vi "MainRunExp.vi"() -> ()   [LabVIEW 2019, in "MotorPID.lvlib"]
uses:
  MotorPID.lvlib
  RunState.ctl
  <vilib>/Platform/TimedLoop/XDataNode/timing_clust.ctl
  <vilib>/Platform/TimedLoop/XDataNode/nitl_modes.ctl
  <vilib>/Platform/TimedLoop/XDataNode/wakeup.ctl
  <vilib>/myRIO/Common/Instrument Driver Framework/myRIO v1.0/UART/vis/myRIO v1.0 Close UART.vi
  <vilib>/addons/control/pid/pid.llb/PID (DBL).vi
  <vilib>/myRIO/Common/Instrument Driver Framework/Utilities/vis/FPGA Ref Manager.vi
  <vilib>/myRIO/Common/Instrument Driver Framework/myRIO v1.0/myRIO v1.0 Reset FPGA.vi
  <vilib>/myRIO/Common/Instrument Driver Framework/myRIO v1.0/IRQ/vis/myRIO v1.0 IRQ Info FGV.vi
  <vilib>/myRIO/Common/Instrument Driver Framework/myRIO v1.0/IRQ/vis/myRIO v1.0 Timer IRQ Info FGV.vi
  <vilib>/myRIO/Common/Instrument Driver Framework/myRIO v1.0/IRQ/vis/myRIO v1.0 ISR Agent.vi
  <vilib>/myRIO/Instrument Drivers/Utilities/vis/Reset Index.vi
  <vilib>/myRIO/Common/Instrument Driver Framework/myRIO v1.0/Resource Manager/vis/myRIO v1.0 Block Write Resource Manager.vi
  <vilib>/Platform/TimedLoop/XDataNode/XDataNode.xnode
  <vilib>/myRIO/Instrument Drivers/Utilities/Utilities.lvlib
  <vilib>/addons/control/pid/NI_PID_pid.lvlib
  <vilib>/Platform/TimedLoop/XDataNode/XDNodeRunTimeDep.lvlib
  <vilib>/ptbypt/NI_PtbyPt.lvlib
panel:
  out "State":u16(ring) items=["StickReset", "MotorReset", "MotorHome", "RunUp", "Runing", "Exit"]
  out "Waveform Chart":T1(graph)
  in  "Setpoint(deg)":dbl(knob) scale=80.0..-80.0
  out "error out":errorcluster
  out "Position(deg)":dbl(knob) scale=80.0..-80.0
  in  "Reset":bool
  in  "Stop Button":bool
  out "MotorResetPOS":dbl[](array[numeric])
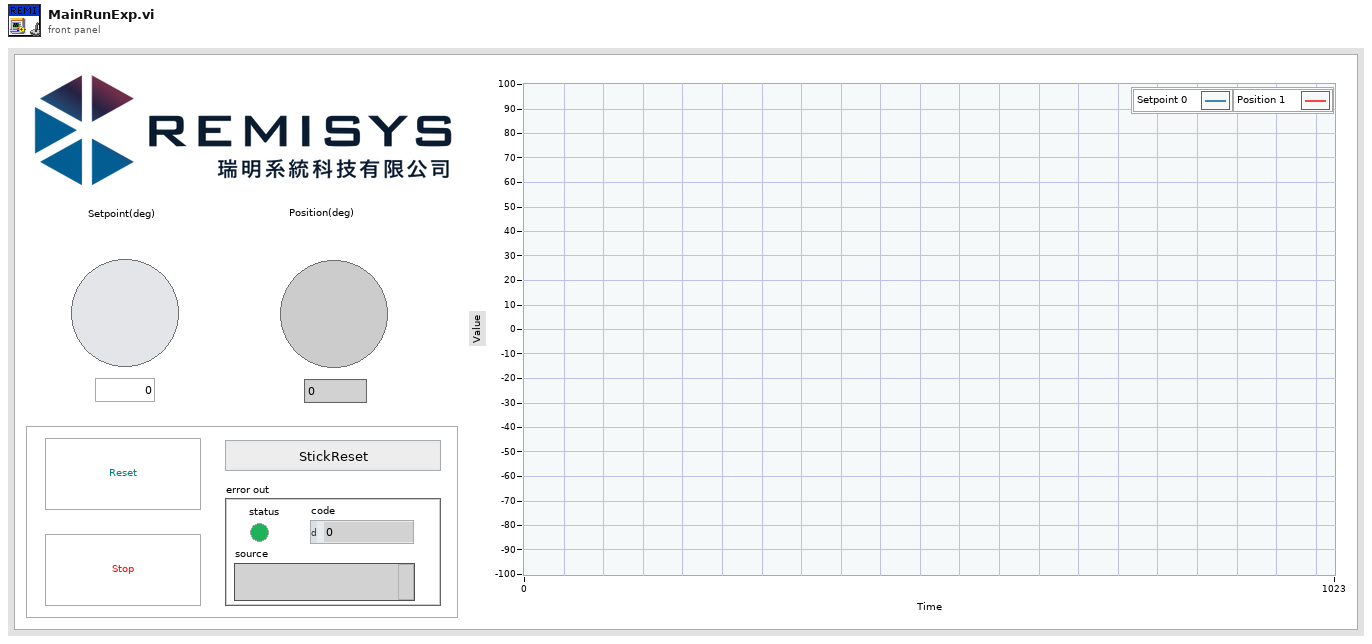
[diagram p1: front panel]
types:
  T1 = cluster{"Setpoint(deg)":dbl, "PresentPOS(deg)":dbl}
  T2 = typedef "MotorPID.lvlib/RunState.ctl" = enum16{"StickReset", "MotorReset", "MotorHome", "RunUp", "Runing", "Exit"}
  T3 = typedef "XDNodeRunTimeDep.lvlib/timing_clust.ctl" = cluster{"Expected End [f-1]":u64, "Actual End [f-1]":u64, "Finished Late? [f-1]":bool, "Expected End [i-1]":u64, "Actual End [i-1]":u64, "Finished Late? [i-1]":bool, "Expected Start [i]":u64, "Actual Start [i]":u64, "Expected Start [f]":u64, "Actual Start [f]":u64, "Source Name":string, "Structure Name":string, "Period":i64, "Deadline":i64, "Offset":i64, "Start":i64, "Priority":i32, "Timeout":i32, "Mode":T4, "Wakeup Reason":T5, "Error":errorcluster, "Source Type":string, "Secondary Source Type":string, "Global End Time":u64, "Global Start Time":u64, "Frame Duration":u64, "Iteration Duration":u64, "Assigned CPU":i32, "I/O Scan Engine Mode":u32}
  T4 = typedef "XDNodeRunTimeDep.lvlib/nitl_modes.ctl" = enum32{"No Change", "Process missed periods, maintain original phase", "Discard missed periods, maintain original phase", "Process missed periods, ignore original phase", "Discard missed periods, ignore original phase"}
  T5 = typedef "XDNodeRunTimeDep.lvlib/wakeup.ctl" = enum32{"Normal", "Aborted", "Asynchronous wakeup", "Timing source error", "Timed loop error", "Timeout"}
  T6 = cluster{"proportional gain (Kc)":dbl, "integral time (Ti, min)":dbl, "derivative time (Td, min)":dbl}
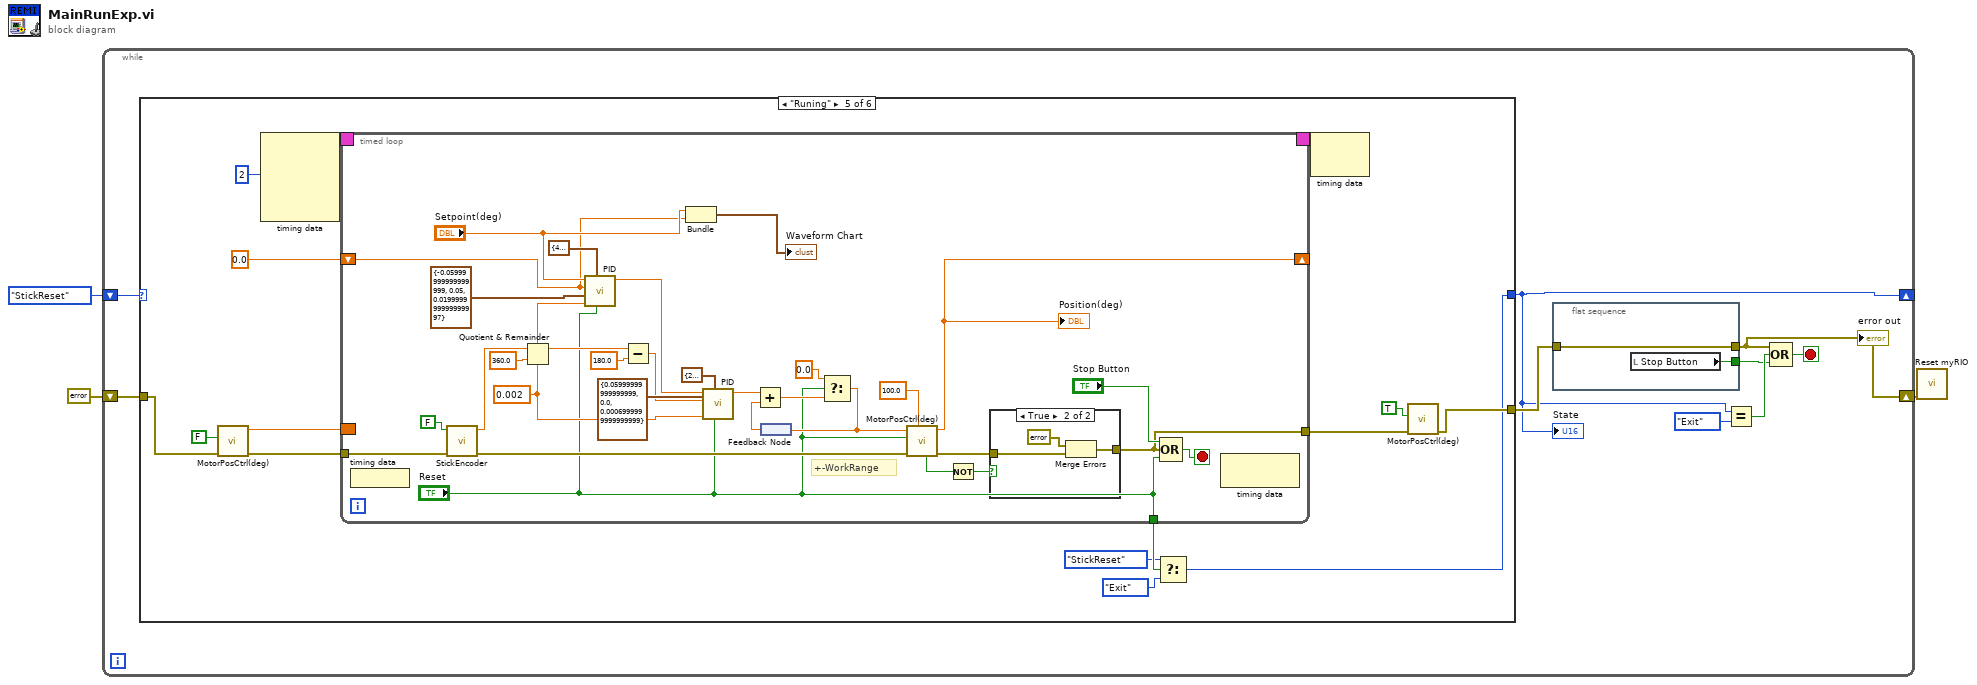
[diagram p0: block diagram]
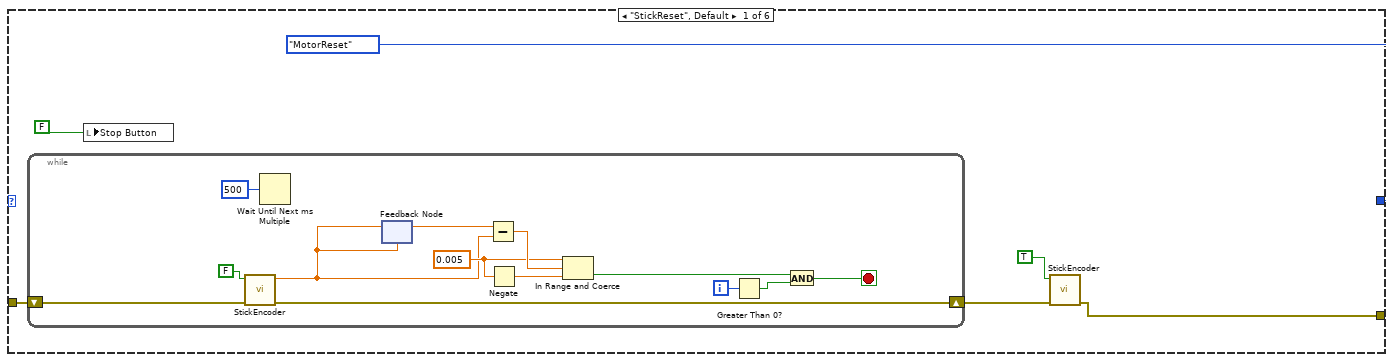
[diagram p2: hidden frame]
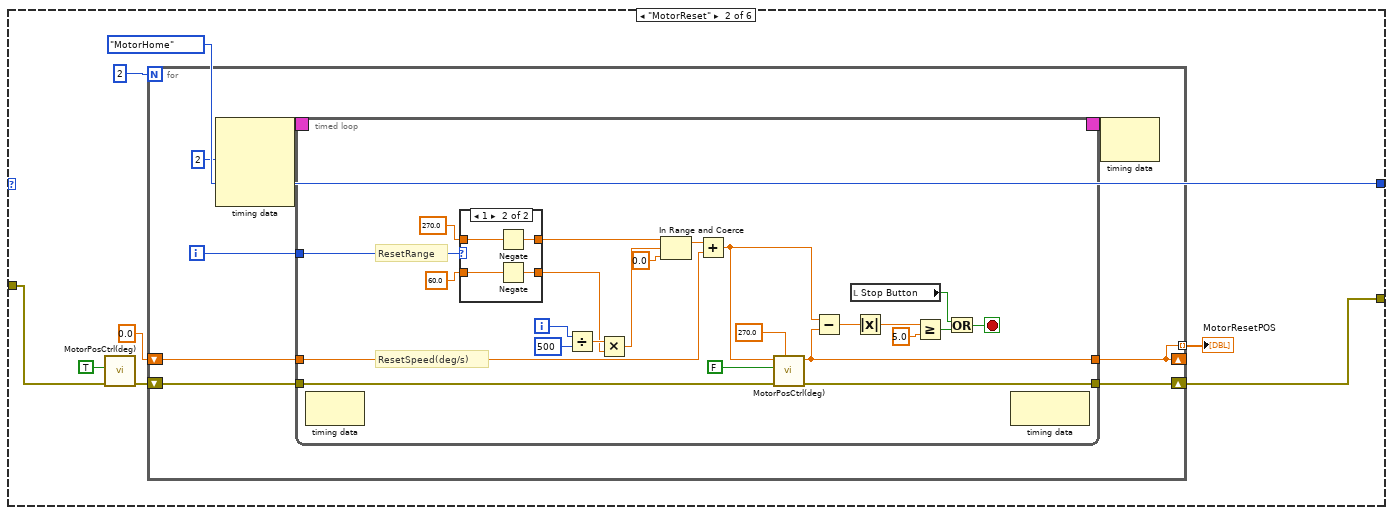
[diagram p3: hidden frame]
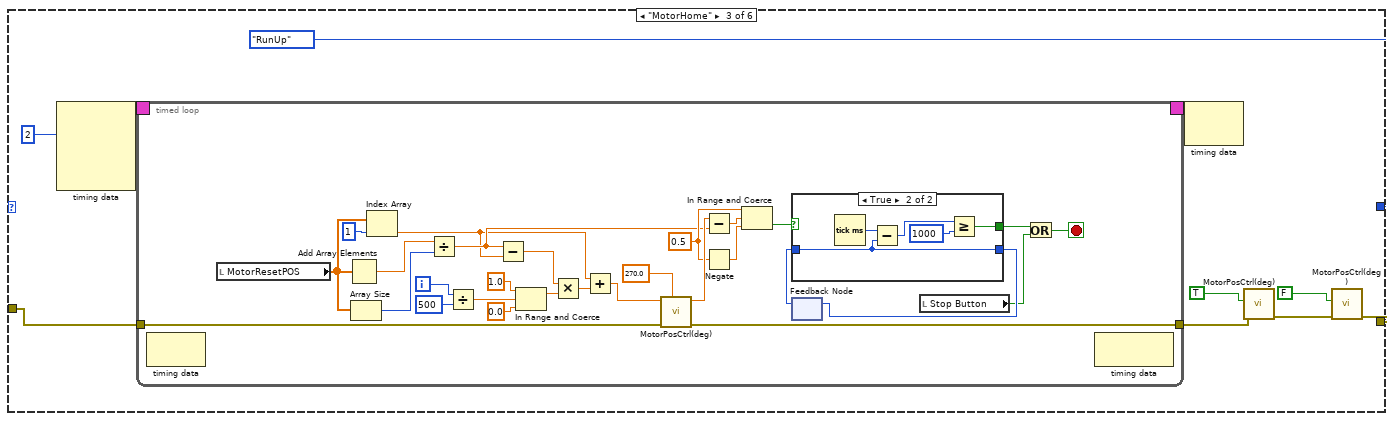
[diagram p5: hidden frame]
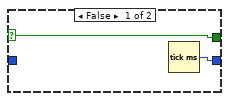
[diagram p6: hidden frame]
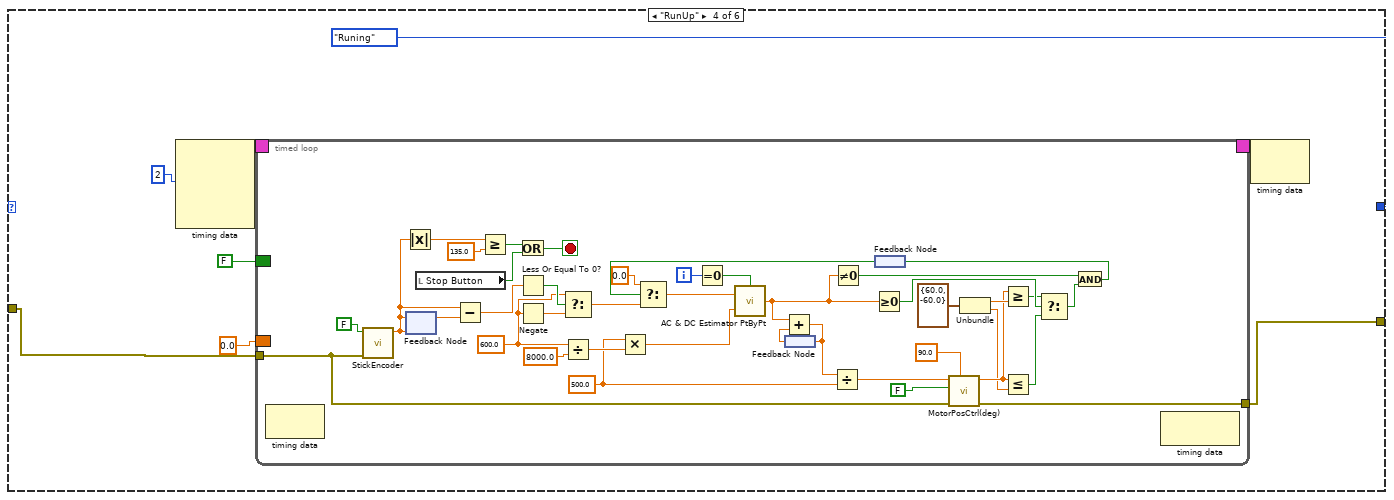
[diagram p7: hidden frame]
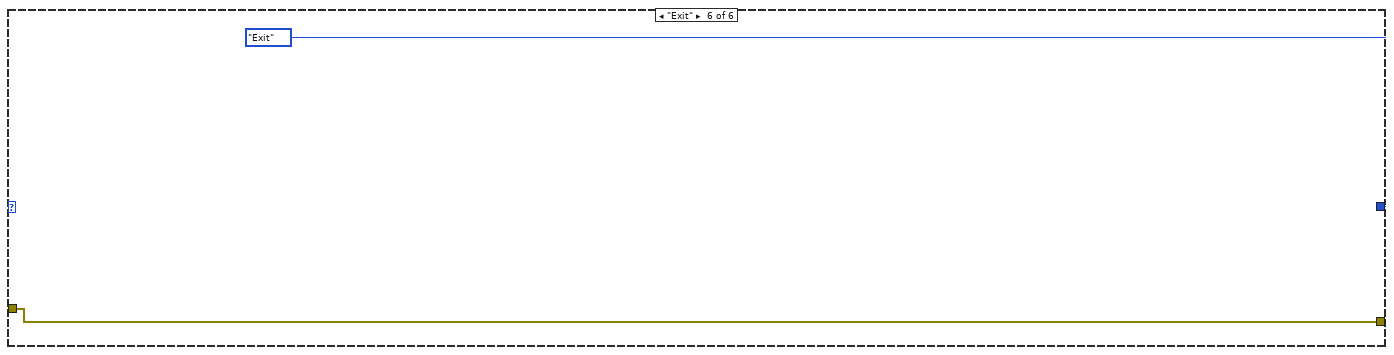
[diagram p9: hidden frame]
diagram:
  n1 = while {
    shift-right: [w5] -> _
    shift-left: RunState."StickReset" -> [w12]
    shift-right: [w4] -> w1
    shift-left: errorcluster {"status"=FALSE, "code"=0, "source"=""} ("error in (no error)") -> [w11]
    stop <- w8 stop-if-true
    n2 = case shown="\"Runing\"" w12 {
      tunnel: w11 -> [w18 w40 w92 w141 w201 w248]
      tunnel: [w17 w41 w86 w139 w195 w248] -> w7
      tunnel: [RunState."MotorReset" RunState."MotorHome" RunState."RunUp" RunState."Runing" w191 RunState."Exit"] -> w5
      frame "StickReset", Default {
        n3 = while {
          shift-right: [w33] -> w20
          shift-left: w18 -> [w32]
          i -> [w26]
          stop <- w23 stop-if-true
          w28 = 0.005 ("upper limit")
          n4 = call "StickEncoder.vi"("error in (no error)"=w32, "Reset Counter"=FALSE) -> ("error out"=w33:errorcluster, "PresentPOS(deg)"=w21:dbl)  [unwired: 8 in]
          n5 = Wait Until Next ms Multiple(millisecond multiple=u32 500) -> ()  [unwired: 1 out]
          n6 = feedback-in #1(w21) -> ()
          n7 = feedback #1(w21) -> (w30:dbl)
          n8 = Subtract(x=w30, y=w21) -> (x-y=w29:dbl)
          n9 = Negate(x=w28) -> (-x=w27:dbl)
          n10 = In Range and Coerce(upper limit=w28, x=w29, lower limit=w27) -> (In Range?=w25:bool)  [unwired: 1 out]
          n11 = Greater Than 0?(x=w26) -> (x > 0?=w24:bool)
          n12 = And(x=w25, y=w24) -> (x .and. y?=w23:bool)
        }
        n13 = local write "Stop Button"(FALSE ("Stop Button")) -> ()
        n14 = call "StickEncoder.vi"("error in (no error)"=w20, "Reset Counter"=TRUE) -> ("error out"=w17:errorcluster)  [unwired: 8 in, 1 out]
      }
      frame "MotorReset" {
        n15 = call "MotorPosCtrl(deg).vi"("error in (no error)"=w40, "Reset Button"=TRUE) -> ("error out"=w39:errorcluster)  [unwired: 6 in, 3 out]
        n16 = for {
          N: 2 -> [_]
          shift-right: [w46] -> w41
          shift-left: w39 -> [w45]
          shift-right: [w42] -> _
          shift-left: 0.0 ("PresentPOS(deg)") -> [w43]
          tunnel: [w42] -> w35 mode=indexing
          i -> [w44]
          n17 = node-c288(i64 2 ("Period")) -> (w49:T3)  [unwired: 3 in]
          n18 = timed-loop {
            timing: w49 -> [_]
            timing-out: [_] -> w48
            tunnel: w45 -> [w50]
            tunnel: [w73] -> w46
            tunnel: w44 -> [w68]
            tunnel: [w56] -> w42
            tunnel: w43 -> [w65]
            i -> [w72]
            stop <- w60 stop-if-true
            # "ResetRange"
            # "ResetSpeed(deg/s)"
            n19 = node-c288() -> ()  [unwired: 1 in, 1 out]
            n20 = case shown="1" w68 {
              tunnel: [w75 w78] -> w67
              tunnel: [w74 w76] -> w63
              tunnel: 270.0 ("Target(deg)") -> [w75 w79]
              tunnel: 60.0 ("y") -> [w74 w77]
              frame 0, Default {
              }
              frame 1 {
                n21 = Negate(x=w79) -> (-x=w78:dbl)
                n22 = Negate(x=w77) -> (-x=w76:dbl)
              }
            }
            n23 = Divide(x=w72, y=500) -> (x/y=w71:dbl)
            n24 = Multiply(x=w71, y=w63) -> (x*y=w70:dbl)
            n25 = In Range and Coerce(upper limit=w67, x=w70, lower limit=0.0) -> (coerced(x)=w66:dbl)  [unwired: 1 out]
            n26 = Add(x=w66, y=w65) -> (x+y=w57:dbl)
            n27 = call "MotorPosCtrl(deg).vi"("WorkRange"=270.0, "error in (no error)"=w50, "Reset Button"=FALSE, "Target(deg)"=w57) -> ("error out"=w73:errorcluster, "PresentPOS(deg)"=w56:dbl)  [unwired: 4 in, 2 out]
            n28 = Subtract(x=w57, y=w56) -> (x-y=w54:dbl)
            n29 = local read "Stop Button"() -> (w59:bool)
            n30 = Absolute Value(x=w54) -> (abs(x)=w53:dbl)
            n31 = Greater Or Equal?(x=w53, y=5.0) -> (x >= y?=w52:bool)
            n32 = Or(x=w59, y=w52) -> (x .or. y?=w60:bool)
            n33 = node-c288() -> ()  [unwired: 1 in, 1 out]
          }
          n34 = node-c288(w48) -> ()  [unwired: 1 out]
        }
        "MotorResetPOS" <- w35
      }
      frame "MotorHome" {
        n35 = node-c288(i64 2 ("Period")) -> (w94:T3)  [unwired: 3 in]
        n36 = timed-loop {
          timing: w94 -> [_]
          timing-out: [_] -> w93
          tunnel: w92 -> [w123]
          tunnel: [w117] -> w90
          i -> [w111]
          stop <- w97 stop-if-true
          w119 = 0.5
          n37 = node-c288() -> ()  [unwired: 1 in, 1 out]
          n38 = local read "MotorResetPOS"() -> (w106:dbl[])
          n39 = Add Array Elements(numeric array=w106) -> (sum=w105:dbl)
          n40 = Array Size(array=w106) -> (size(s)=w122:i32)
          n41 = Index Array(array=w106, index=1) -> (element=w100:dbl)
          n42 = Divide(x=w105, y=w122) -> (x/y=w102:dbl)
          n43 = Divide(x=w111, y=500) -> (x/y=w109:dbl)
          n44 = Subtract(x=w102, y=w100) -> (x-y=w101:dbl)
          n45 = In Range and Coerce(upper limit=1.0, x=w109, lower limit=0.0) -> (coerced(x)=w104:dbl)  [unwired: 1 out]
          n46 = Multiply(x=w101, y=w104) -> (x*y=w103:dbl)
          n47 = Add(x=w100, y=w103) -> (x+y=w99:dbl)
          n48 = call "MotorPosCtrl(deg).vi"("WorkRange"=270.0, "error in (no error)"=w123, "Target(deg)"=w99) -> ("error out"=w117:errorcluster, "PresentPOS(deg)"=w121:dbl)  [unwired: 5 in, 2 out]
          n49 = Subtract(x=w121, y=w102) -> (x-y=w120:dbl)
          n50 = Negate(x=w119) -> (-x=w118:dbl)
          n51 = In Range and Coerce(upper limit=w119, x=w120, lower limit=w118) -> (In Range?=w112:bool)  [unwired: 1 out]
          n52 = feedback #2() -> (w115:u32)  [unwired: 1 in]
          n53 = case shown="True" w112 {
            selector: w112 -> [w124 _]
            tunnel: [w125 w126] -> w116
            tunnel: w115 -> [_ w126]
            tunnel: [w124 w127] -> w113
            frame False {
              n54 = Tick Count (ms)() -> (millisecond timer value=w125:u32)
            }
            frame True {
              n55 = Tick Count (ms)() -> (millisecond timer value=w130:u32)
              n56 = Subtract(x=w130, y=w126) -> (x-y=w129:u32)
              n57 = Greater Or Equal?(x=w129, y=u32 1000) -> (x >= y?=w127:bool)
            }
          }
          n58 = feedback-in #2(w116) -> ()
          n59 = local read "Stop Button"() -> (w114:bool)
          n60 = Or(x=w113, y=w114) -> (x .or. y?=w97:bool)
          n61 = node-c288() -> ()  [unwired: 1 in, 1 out]
        }
        n62 = node-c288(w93) -> ()  [unwired: 1 out]
        n63 = call "MotorPosCtrl(deg).vi"("error in (no error)"=w90, "Reset Button"=TRUE) -> ("error out"=w87:errorcluster)  [unwired: 6 in, 3 out]
        n64 = call "MotorPosCtrl(deg).vi"("error in (no error)"=w87, "Reset Button"=FALSE) -> ("error out"=w86:errorcluster)  [unwired: 6 in, 3 out]
      }
      frame "RunUp" {
        n65 = node-c288(i64 2 ("Period")) -> (w144:T3)  [unwired: 3 in]
        n66 = timed-loop {
          timing: w144 -> [_]
          timing-out: [_] -> w143
          tunnel: w141 -> [w182]
          tunnel: [w177] -> w139
          border: 0.0 ("PresentPOS(deg)") -> [_]
          border: FALSE -> [_]
          i -> [w184]
          stop <- w174 stop-if-true
          w170 = 600.0 ("MaxSpeed(deg/s)")
          w160 = 500.0 ("x")
          n67 = node-c288() -> ()  [unwired: 1 in, 1 out]
          n68 = call "StickEncoder.vi"("error in (no error)"=w182, "Reset Counter"=FALSE) -> ("PresentPOS(deg)"=w147:dbl)  [unwired: 8 in, 1 out]
          n69 = Absolute Value(x=w147) -> (abs(x)=w179:dbl)
          n70 = feedback-in #3(w147) -> ()
          n71 = feedback #3(w147) -> (w180:dbl)
          n72 = local read "Stop Button"() -> (w176:bool)
          n73 = Subtract(x=w147, y=w180) -> (x-y=w173:dbl)
          n74 = Greater Or Equal?(x=w179, y=135.0) -> (x >= y?=w175:bool)
          n75 = Or(x=w175, y=w176) -> (x .or. y?=w174:bool)
          n76 = Less Or Equal To 0?(x=w173) -> (x <= 0?=w172:bool)
          n77 = Negate(x=w170) -> (-x=w171:dbl)
          n78 = Select(t=w170, s=w172, f=w171) -> (s? t:f=w164:dbl)
          n79 = Divide(x=w170, y=8000.0 ("Acc(deg/ss)")) -> (x/y=w169:dbl)
          n80 = Multiply(x=w160, y=w169) -> (x*y=w146:dbl)
          n81 = Equal To 0?(x=w184) -> (x = 0?=w183:bool)
          n82 = feedback #4() -> (w167:dbl)
          n83 = feedback #5() -> (w165:bool)
          n84 = Select(t=0.0, s=w165, f=w164) -> (s? t:f=w162:dbl)
          n85 = call <vilib>:"AC & DC Estimator PtByPt.vi"("signal"=w162, "sample length"=w146, "initialize"=w183) -> ("DC estimate (V)"=w151:dbl)  [unwired: 2 out]
          n86 = Add(x=w151, y=w167) -> (x+y=w161:dbl)
          n87 = feedback-in #4(w161) -> ()
          n88 = Divide(x=w161, y=w160) -> (x/y=w159:dbl)
          n89 = Not Equal To 0?(x=w151) -> (x != 0?=w150:bool)
          n90 = Greater Or Equal To 0?(x=w151) -> (x >= 0?=w157:bool)
          n91 = call "MotorPosCtrl(deg).vi"("WorkRange"=90.0, "error in (no error)"=w182, "Reset Button"=FALSE, "Target(deg)"=w159) -> ("error out"=w177:errorcluster, "PresentPOS(deg)"=w155:dbl)  [unwired: 4 in, 2 out]
          n92 = Unbundle(cluster{"UpLimit":dbl, "DownLimit":dbl} {"UpLimit"=60.0, "DownLimit"=-60.0} ("RunUpLimuit")) -> ("UpLimit"=w156:dbl, "DownLimit"=w154:dbl)
          n93 = Greater Or Equal?(x=w155, y=w156) -> (x >= y?=w153:bool)
          n94 = Less Or Equal?(x=w155, y=w154) -> (x <= y?=w152:bool)
          n95 = Select(t=w153, s=w157, f=w152) -> (s? t:f=w149:bool)
          n96 = And(x=w150, y=w149) -> (x .and. y?=w148:bool)
          n97 = feedback-in #5(w148) -> ()
          n98 = node-c288() -> ()  [unwired: 1 in, 1 out]
        }
        n99 = node-c288(w143) -> ()  [unwired: 1 out]
      }
      frame "Runing" {
        n100 = call "MotorPosCtrl(deg).vi"("error in (no error)"=w201, "Reset Button"=FALSE) -> ("error out"=w200:errorcluster, "PresentPOS(deg)"=w198:dbl)  [unwired: 6 in, 2 out]
        n101 = node-c288(i64 2 ("Period")) -> (w205:T3)  [unwired: 3 in]
        n102 = timed-loop "Timed Loop" {
          tunnel: [w211] -> w197
          timing: w205 -> [_]
          timing-out: [_] -> w204
          border: w198 -> [_]
          shift-right: [w209] -> _
          shift-left: 0.0 -> [w207]
          tunnel: w200 -> [w221]
          tunnel: ["Reset"] -> w194
          stop <- w212 stop-if-true
          w227 = 0.002 ("dt (s)")
          # "+-WorkRange"
          n103 = node-c288() -> ()  [unwired: 1 in]
          n104 = call "StickEncoder.vi"("error in (no error)"=w221, "Reset Counter"=FALSE) -> ("error out"=w235:errorcluster, "PresentPOS(deg)"=w219:dbl)  [unwired: 8 in]
          n105 = Quotient & Remainder(x=w219, y=360.0) -> (x-y*floor(x/y)=w218:dbl)  [unwired: 1 out]
          n106 = call-poly <vilib>:"PID.vi"("reinitialize? (F)"="Reset", "output range"=cluster{"output high":dbl, "output low":dbl} {"output high"=45.0, "output low"=-45.0}, "dt (s)"=w227, "PID gains"=T6 {"proportional gain (Kc)"=-0.05999999999999999, "integral time (Ti, min)"=0.05, "derivative time (Td, min)"=0.019999999999999997} ("PID gains 2"), "process variable"=w207, "setpoint"="Setpoint(deg)") -> ("output"=w222:dbl)  [unwired: 4 in, 1 out]
          n107 = Subtract(x=w218, y=180.0) -> (x-y=w226:dbl)
          n108 = Bundle("Setpoint(deg)"="Setpoint(deg)", w207) -> (→"Waveform Chart":cluster{"Setpoint(deg)":dbl, dbl})  [unwired: 1 in]
          n109 = call-poly <vilib>:"PID.vi"("reinitialize? (F)"="Reset", "output range"=cluster{"output high":dbl, "output low":dbl} {"output high"=2.0, "output low"=-2.0}, "dt (s)"=w227, "PID gains"=T6 {"proportional gain (Kc)"=0.05999999999999999, "integral time (Ti, min)"=0.0, "derivative time (Td, min)"=0.0006999999999999999}, "process variable"=w226, "setpoint"=w222) -> ("output"=w224:dbl)  [unwired: 4 in, 1 out]
          n110 = feedback #6() -> (w232:dbl)
          n111 = Add(x=w224, y=w232) -> (x+y=w231:dbl)
          n112 = Select(t=0.0, s="Reset", f=w231) -> (s? t:f=w229:dbl)
          n113 = feedback-in #6(w229) -> ()
          n114 = call "MotorPosCtrl(deg).vi"("WorkRange"=100.0, "error in (no error)"=w235, "Reset Button"="Reset", "Target(deg)"=w229) -> ("error out"=w214:errorcluster, "PresentPOS(deg)"=w209:dbl, "In Range?"=w216:bool)  [unwired: 4 in, 1 out]
          "Position(deg)" <- w209
          n115 = Not(x=w216) -> (.not. x?=w215:bool)
          n116 = case shown="True" w215 {
            tunnel: w214 -> [w237 w240]
            tunnel: [w237 w238] -> w211
            frame False {
            }
            frame True {
              n117 = Merge Errors(errorcluster {"status"=TRUE, "code"=10000, "source"="Out of work range "} ("error in (no error)"), w240) -> (w238:errorcluster)
            }
          }
          n118 = Compound Arithmetic op=OR("Stop Button", w211, "Reset") -> (w212:bool)
          n119 = node-c288() -> ()  [unwired: 1 in, 1 out]
        }
        n120 = Select(t=RunState."StickReset", s=w194, f=RunState."Exit") -> (s? t:f=w191:T2)
        n121 = node-c288(w204) -> ()  [unwired: 1 out]
        n122 = call "MotorPosCtrl(deg).vi"("error in (no error)"=w197, "Reset Button"=TRUE) -> ("error out"=w195:errorcluster)  [unwired: 6 in, 3 out]
      }
      frame "Exit" {
      }
    }
    "State" <- w5
    n123 = flat-sequence {
      tunnel: w7 -> [w13]
      tunnel: [w14] -> w6
      tunnel: [w13] -> w4
      frame #0 {
        n124 = local read "Stop Button"() -> (w14:bool)
      }
    }
    n125 = Equal?(x=w5, y=RunState."Exit") -> (x = y?=w9:bool)
    n126 = Compound Arithmetic op=OR(w4, w9, w6) -> (w8:bool)
    "error out" <- w4
  }
  n127 = call <vilib>:"Reset myRIO.vi"("error in (no error)"=w1) -> ()  [unwired: 10 in, 1 out]
